vi "Begin.vi"(8 "error in (no error)":errorcluster, 10 "Settings In":variant, 11 "Demo Mode in":refnum<class "Demo Mode.lvclass">) -> (0 "error out":errorcluster, 3 "Demo Mode out":refnum<class "Demo Mode.lvclass">)   [LabVIEW 2019, in "Joysticks.lvlib" / "Demo Mode.lvclass"]
doc: "This VI is used to open the joystick control references."
uses:
  Demo Mode.lvclass
  Joysticks.lvclass
  <vilib>/Rock Robotics/WPI/Joystick/WPI_JoystickDeviceEnum.ctl
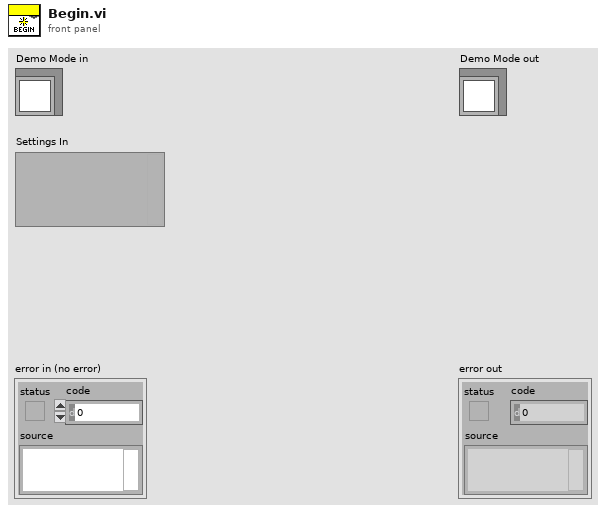
[diagram p1: front panel]
types:
  T1 = typedef "WPI_JoystickDeviceEnum.ctl" = enum16{"USB 0", "USB 1", "USB 2", "USB 3", "USB 4", "USB 5"}
  T2 = typedef "WPI_JoystickDevRef.ctl" = cluster{"Device":T1}
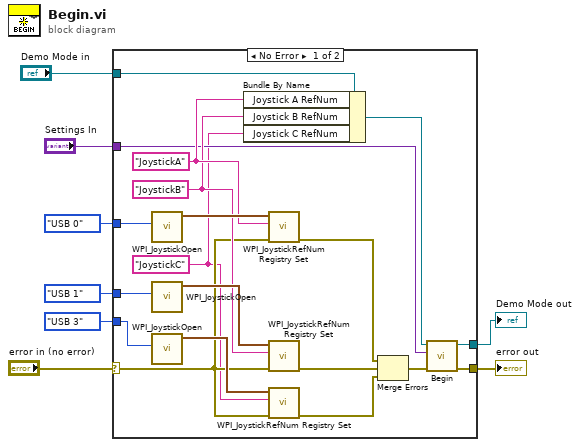
[diagram p0: block diagram]
diagram:
  n1 = case shown="No Error" "error in (no error)" {
    selector: "error in (no error)" -> [w14 w29]
    tunnel: [w27 w29] -> w3
    tunnel: [w26 w28] -> w5
    tunnel: "Demo Mode in" -> [w25 w28]
    tunnel: WPI_JoystickDeviceEnum."USB 0" ("JoystickDevice") -> [w22 _]
    tunnel: WPI_JoystickDeviceEnum."USB 1" ("JoystickDevice") -> [w21 _]
    tunnel: "Settings In" -> [w17 _]
    tunnel: WPI_JoystickDeviceEnum."USB 3" ("JoystickDevice") -> [w15 _]
    frame No Error {
      w9 = "JoystickC" ("Joystick B RefNum")
      w18 = "JoystickB" ("Joystick B RefNum")
      w19 = "JoystickA" ("Joystick A RefNum")
      n2 = call <vilib>:"WPI_JoystickOpen.vi"("JoystickDevice"=w22) -> ("JoystickDevRef"=w23:T2)  [unwired: 10 in]
      n3 = call <vilib>:"WPI_JoystickOpen.vi"("JoystickDevice"=w21) -> ("JoystickDevRef"=w24:T2)  [unwired: 10 in]
      n4 = call <vilib>:"WPI_JoystickOpen.vi"("JoystickDevice"=w15) -> ("JoystickDevRef"=w16:T2)  [unwired: 10 in]
      n5 = Bundle By Name(cluster=w25, "Joystick A RefNum"=w19, "Joystick B RefNum"=w18, "Joystick C RefNum"=w9) -> (w20:refnum<class "Demo Mode.lvclass">)
      n6 = call <vilib>:"WPI_JoystickRefNum Registry Set.vi"("error in (no error)"=w14, "refnum name"=w19, "JoystickDevRef"=w23) -> ("error out"=w12:errorcluster)  [unwired: 7 in, 1 out]
      n7 = call <vilib>:"WPI_JoystickRefNum Registry Set.vi"("error in (no error)"=w14, "refnum name"=w18, "JoystickDevRef"=w24) -> ("error out"=w11:errorcluster)  [unwired: 7 in, 1 out]
      n8 = call <vilib>:"WPI_JoystickRefNum Registry Set.vi"("error in (no error)"=w14, "refnum name"=w9, "JoystickDevRef"=w16) -> ("error out"=w10:errorcluster)  [unwired: 7 in, 1 out]
      n9 = Merge Errors(w12, w11, w10) -> (w13:errorcluster)
      n10 = call-parent "Begin.vi"("error in (no error)"=w13, "Settings In"=w17, "Joysticks in"=w20) -> ("error out"=w27:errorcluster, "Joysticks out"=w26:refnum<class "Demo Mode.lvclass">)  [unwired: 7 in]
    }
    frame Error {
    }
  }
  "error out" <- w3
  "Demo Mode out" <- w5
